vi "Write TagDistanceArray.vi"(8 "error in (no error)":errorcluster, 10 "TagDistanceArray":T1(array[cluster]), 11 "Anchor in":refnum<class "Anchor.lvclass">) -> (0 "error out":errorcluster, 3 "Anchor out":refnum<class "Anchor.lvclass">)   [LabVIEW 2014, in "Anchor.lvclass"]
doc: "This VI writes data to anchor class. The data is a Tag object plus its \nmeasured distance from the Anchor object."
uses:
  Anchor.lvclass
  Tag.lvclass
  Anchor.lvclass/Anchor.ctl
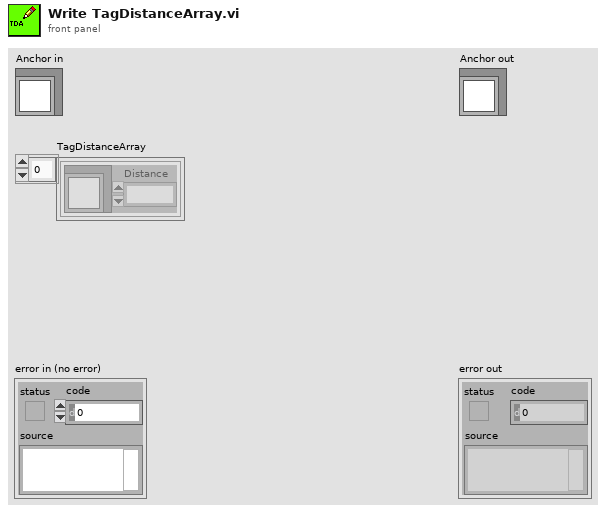
[diagram p1: front panel]
types:
  T1 = cluster{"Tag.lvclass":refnum<class "Tag.lvclass">, "Distance":dbl}[]
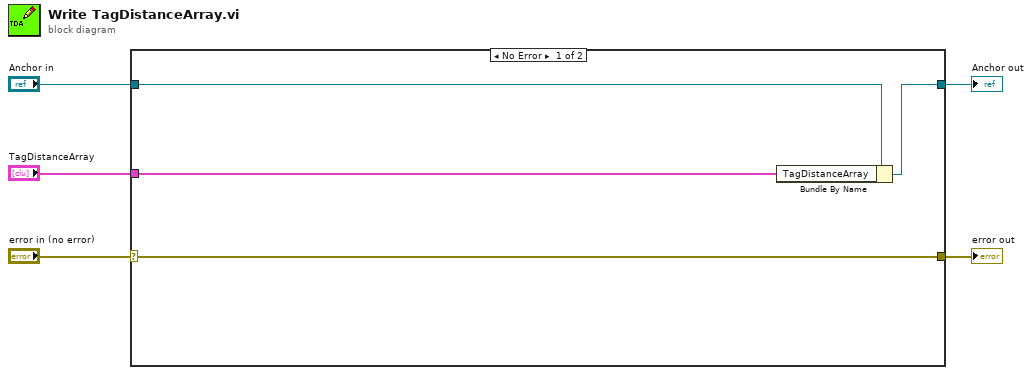
[diagram p0: block diagram]
diagram:
  n1 = case shown="No Error" "error in (no error)" {
    selector: "error in (no error)" -> [w9 w10]
    tunnel: [w9 w10] -> w4
    tunnel: [w8 w11] -> w2
    tunnel: "Anchor in" -> [w7 w11]
    tunnel: "TagDistanceArray" -> [w6 _]
    frame No Error {
      n2 = Bundle By Name(cluster=w7, "TagDistanceArray"=w6) -> (w8:refnum<class "Anchor.lvclass">)
    }
    frame Error {
    }
  }
  "error out" <- w4
  "Anchor out" <- w2
